vi "Write Timestamp(1).vi"() -> ()   [LabVIEW 2021]
panel:
  in  "Error in (no error)":errorcluster
  out "Error out":errorcluster
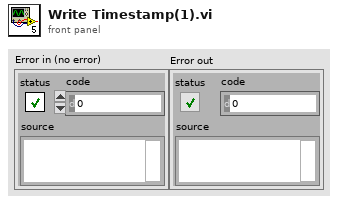
[diagram p1: front panel]
types:
  T1 = enum32{"Invalid", "Standard", "Closed", "Hidden", "Minimized", "Maximized"}
  T2 = enum16{"open", "replace", "create", "open or create", "replace or create", "replace or create with confirmation"}
  T3 = typedef "Paths.ctl" = cluster{"Configuration":path, "Event Logs":path, "Error Logs":path, "Macros":path, "Camera Settings":path, "Settings.ini":path, "UserInfo.bin":path, "TimeStamp File":path, "FileCounter.txt":path, "FFC Images":path, "Calibration.txt":path, "Bright Images - FFC":path, "Dark Images - FFC":path, "Last FFC Time File":path, "BG Subtraction Folder":path, "BG Mask":path, "LUTs Folder":path}
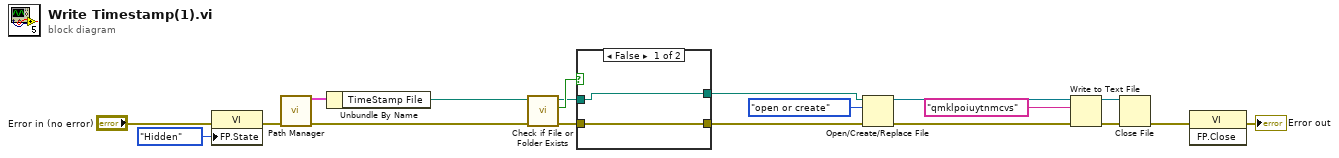
[diagram p0: block diagram]
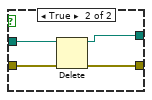
[diagram p2: hidden frame]
diagram:
  n1 = property class="VI"(error in="Error in (no error)", "FP.State"=T1."Hidden" ("Front Panel Window:State")) -> (error out=w8:errorcluster)  [unwired: 1 in, 1 out]
  n2 = call "Path Manager.vi"("error in (no error)"=w8) -> ("Cluster"=w19:T3, "Error out"=w6:errorcluster)  [unwired: 13 in]
  n3 = Unbundle By Name(w19) -> ("TimeStamp File"=w7:path)
  n4 = call <vilib>:"Check if File or Folder Exists.vi"("error in (no error)"=w6, "path"=w7) -> ("error out"=w4:errorcluster, "file or folder exists?"=w5:bool, "dup path"=w2:path)  [unwired: 7 in]
  n5 = case shown="False" w5 {
    tunnel: w4 -> [w20 w25]
    tunnel: [w20 w24] -> w3
    tunnel: w2 -> [w21 w23]
    tunnel: [w21 w22] -> w1
    frame False {
    }
    frame True {
      n6 = Delete(path (use dialog)=w23, error in=w25) -> (deleted path=w22:path, error out=w24:errorcluster)  [unwired: 3 in, 1 out]
    }
  }
  n7 = Open/Create/Replace File(file path (use dialog)=w1, error in=w3, operation (0:open)=T2."open or create") -> (refnum out=w16:refnum<file>, error out=w15:errorcluster)  [unwired: 3 in, 1 out]
  n8 = Write to Text File(file (use dialog)=w16, text="qmklpoiuytnmcvs", error in=w15) -> (refnum out=w14:refnum<file>, error out=w13:errorcluster)  [unwired: 1 in, 1 out]
  n9 = Close File(refnum=w14, error in=w13) -> (error out=w12:errorcluster)  [unwired: 1 out]
  n10 = invoke class="VI" method="FP.Close"(error in=w12) -> (error out=→"Error out":errorcluster)  [unwired: 2 in, 2 out]
